vi "test_Set PCL Decimation to 0.vi"(8 "error in (no error)":errorcluster, 11 "TestCase in":refnum<class "Instrument Addon Scripting API Custom Device Unit Tests.lvclass">) -> (0 "error out":errorcluster, 3 "TestCase out":refnum<class "Instrument Addon Scripting API Custom Device Unit Tests.lvclass">)   [LabVIEW 2019, in "Instrument Addon Scripting API Custom Device Unit Tests.lvclass"]
uses:
  Instrument Addon Scripting API Custom Device Unit Tests.lvclass
  Instrument Addon Scripting API Custom Device Unit Tests.lvclass/Instrument Addon Scripting API Custom Device Unit Tests.ctl
  <vilib>/addons/_JKI Toolkits/VI Tester/TestCase.llb/TestCase.lvclass
  APIs/Scripting API/Instrument Addon Scripting API.lvlib
  C:/Program Files (x86)/National Instruments/LabVIEW 2019/vi.lib/addons/_JKI Toolkits/VI Tester/TestCase.llb/TestCase.lvclass
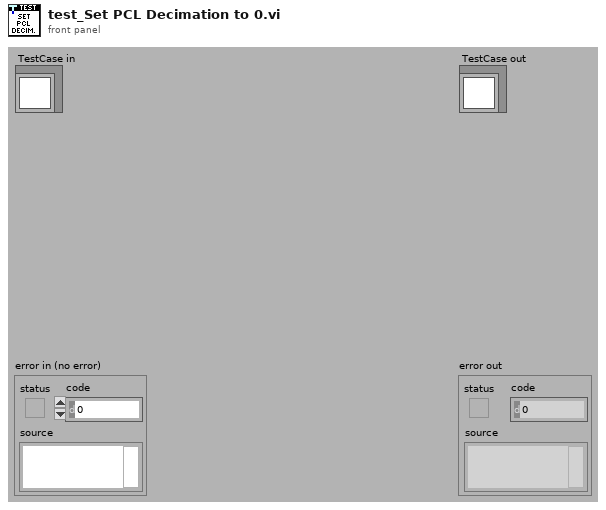
[diagram p1: front panel]
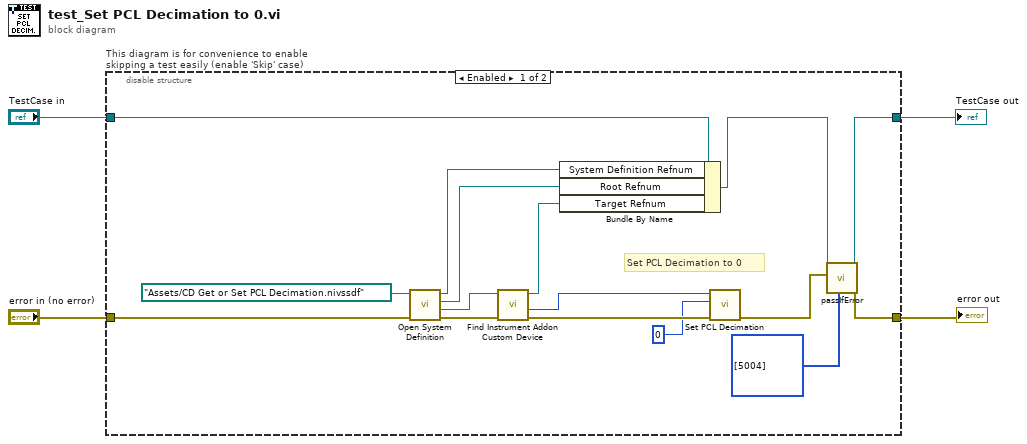
[diagram p0: block diagram]
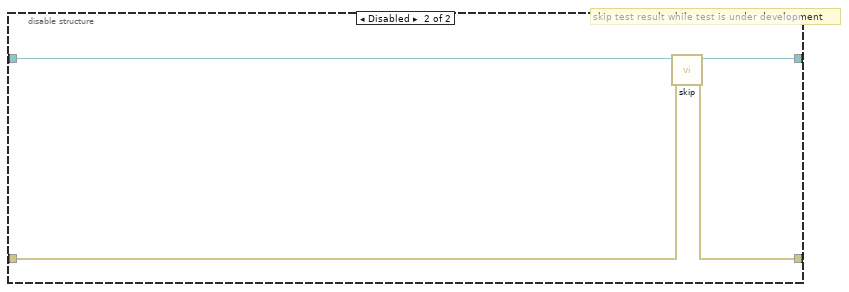
[diagram p2: hidden frame]
diagram:
  n1 = disable-structure "This diagram is for convenience to enable skipping a test easily (enable 'Skip' case)" shown="Enabled" {
    disable-tunnel: "TestCase in" -> [w9 w24]
    disable-tunnel: [w20 w22] -> w1
    disable-tunnel: [w19 w23] -> w3
    disable-tunnel: "error in (no error)" -> [w18 w21]
    frame Enabled {
      # "Set PCL Decimation to 0"
      n2 = call "Open System Definition.vi"("error in (no error)"=w18, "System Definition File"=path "Assets/CD Get or Set PCL Decimation.nivssdf") -> ("error out"=w15:errorcluster, "Target Refnum"=w16:refnum<k24>, "Root Refnum"=w6:refnum<k24>, "System Definition Refnum"=w7:refnum<k24>)  [unwired: 6 in]
      n3 = call "Find Instrument Addon Custom Device.vi"("error in"=w15, "target in"=w16) -> ("error out"=w14:errorcluster, "NodeID"=w12:u64, "target out"=w5:refnum<k24>)  [unwired: 7 in]
      n4 = Bundle By Name(cluster=w9, "System Definition Refnum"=w7, "Root Refnum"=w6, "Target Refnum"=w5) -> (w8:refnum<class "Instrument Addon Scripting API Custom Device Unit Tests.lvclass">)
      n5 = call "Set PCL Decimation.vi"("error in (no error)"=w14, "PCL decimation"=u32 0 ("PCL Decimation"), "instrument addon refnum in"=w12) -> ("error out"=w10:errorcluster)  [unwired: 7 in, 1 out]
      n6 = call-dynamic "passIfError.vi"("passing error codes (default = any error code)"=i32[] [5004], "error"=w10, "TestCase in"=w8) -> ("error out"=w19:errorcluster, "TestCase out"=w20:refnum<class "Instrument Addon Scripting API Custom Device Unit Tests.lvclass">)  [unwired: 7 in]
    }
    frame Disabled {
      # "skip test result while test is under development"
      n7 = call <vilib>:"skip.vi"("error in (no error)"=w21, "TestCase in"=w24) -> ("error out"=w23:errorcluster, "TestCase out"=w22:refnum<class "Instrument Addon Scripting API Custom Device Unit Tests.lvclass">)  [unwired: 8 in]
    }
  }
  "error out" <- w3
  "TestCase out" <- w1
